vi "Real world signal (subVI).vi"(8 "error in (no error)":errorcluster, 9 "sampling info":cluster{"Fs":dbl, "#s":dbl}={"Fs"=51200.0, "#s"=1024.0}, 11 "signal generator":T1={"signal type"=enum."Sine Wave", "frequency"=1000.0, "amplitude"=1.0}) -> (0 "error out":errorcluster, 3 "time signal":waveform(dbl))   [LabVIEW 2023]
doc: "This VI simulates a Real world signal. White noise (1mV) is added to a typical test signal (1V) in order to simulate a signal as it could be acquired using a DAQ board."
uses:
  <vilib>/measure/NI_MABase.lvlib
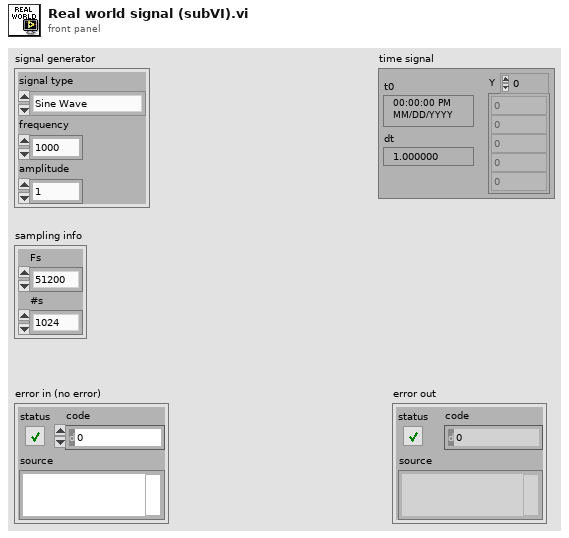
[diagram p1: front panel]
types:
  T1 = cluster{"signal type":enum16{"Sine Wave", "Triangle Wave", "Square Wave", "Sawtooth Wave"}, "frequency":dbl, "amplitude":dbl}
  T2 = enum16{"Sine Wave", "Triangle Wave", "Square Wave", "Sawtooth Wave"}
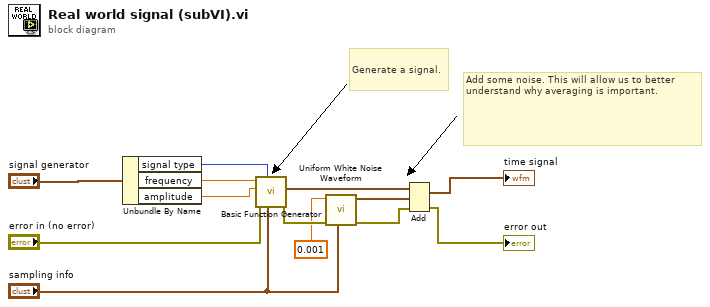
[diagram p0: block diagram]
diagram:
  # "Generate a signal."
  # "Add some noise. This will allow us to better understand why averaging is important."
  n1 = Unbundle By Name("signal generator") -> ("signal type"=w3:T2, "frequency"=w2:dbl, "amplitude"=w1:dbl)
  n2 = call <vilib>:"Basic Function Generator.vi"("sampling info"="sampling info", "signal type"=w3, "error in (no error)"="error in (no error)", "amplitude"=w1, "frequency"=w2) -> ("error out"=w12:errorcluster, "signal out"=w7:waveform(dbl))  [unwired: 4 in, 1 out]
  n3 = call <vilib>:"Uniform White Noise Waveform.vi"("sampling info"="sampling info", "error in (no error)"=w12, "amplitude"=0.001) -> ("error out"=w10:errorcluster, "signal out"=w6:waveform(dbl))  [unwired: 7 in]
  n4 = Add(1:w6, 2:w7, 4:w10) -> (0:→"time signal":waveform(dbl), 3:→"error out":errorcluster)
